vi "Publish Camera Settings.vi"(8 "error in (no error)":errorcluster, 10 "Camera Settings":variant, 11 "IMAQdx Actor in":refnum<class "IMAQdx Actor.lvclass">) -> (0 "error out":errorcluster, 3 "IMAQdx Actor out":refnum<class "IMAQdx Actor.lvclass">)   [LabVIEW 2020, in "IMAQdx Actor.lvlib" / "IMAQdx Actor.lvclass"]
uses:
  IMAQdx Actor.lvclass
  C:/Users/AlexK/work/LabVIEW Programme/POLARIS CAM Log Abw und E/Submodules/HIJ Vision/Camera Actors/Camera Actor/Camera Actor/Camera Actor.lvclass
  IMAQdx Actor.lvclass/IMAQdx Actor.ctl
  Camera Actor/Camera Actor/Camera Actor.lvclass/Camera Actor.ctl
  Camera Actor/Camera Actor/Read Parameter Filter.vi
  Camera Actor/Camera Actor/Camera Actor.lvclass
  <vilib>/vision/driver/NI_Vision_Acquisition_Software.lvlib
  <resource>/objmgr/imaqdx.rc
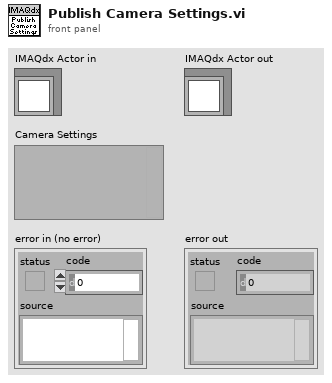
[diagram p1: front panel]
types:
  T1 = typedef "Camera Actor.lvlib/Camera Actor.lvclass/Parameter Filters.ctl" = cluster{"Filter":string[], "Exclude strings":string[]}
  T2 = typedef "IMAQdx.ctl" = refnum<k21>
  T3 = typedef "NI_Vision_Acquisition_Software.lvlib/IMAQdx Attribute Type.ctl" = enum32{"U32", "I64", "DBL", "String", "Enum", "Bool", "Command"}
  T4 = cluster{"Attribute Type":T3, "Readable":bool, "Writable":bool, "Attribute Name":string}[]
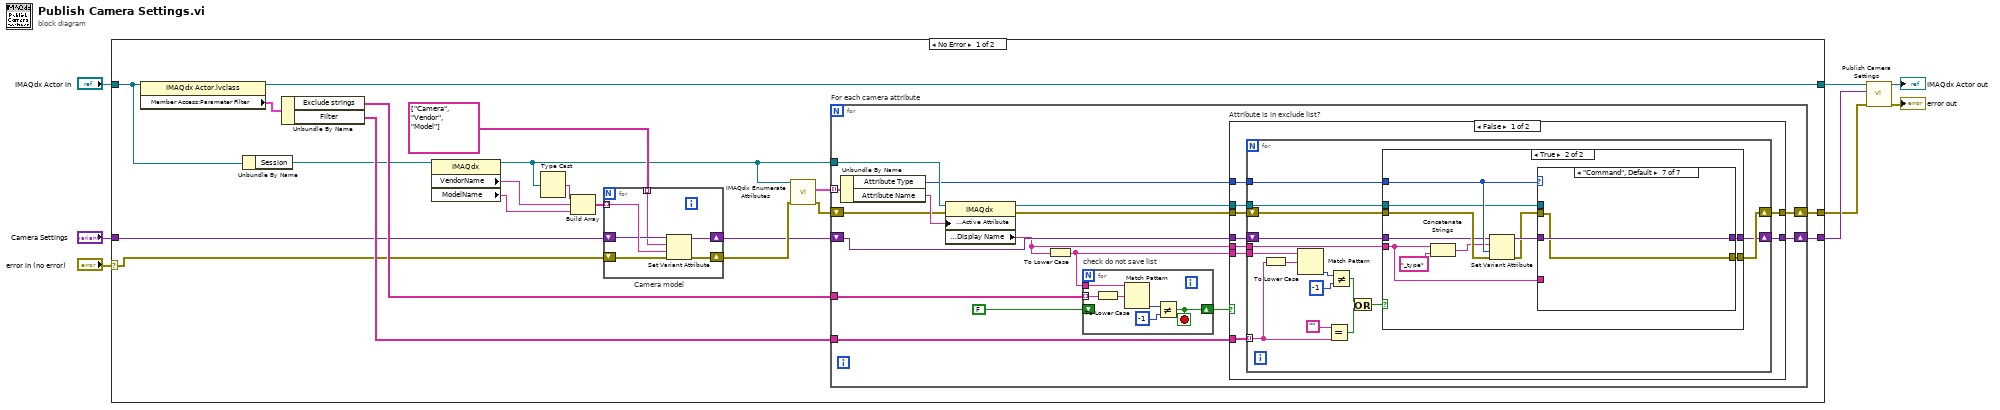
[diagram p0: block diagram]
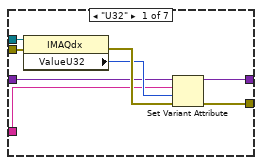
[diagram p3: hidden frame]
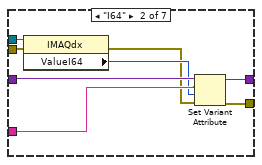
[diagram p4: hidden frame]
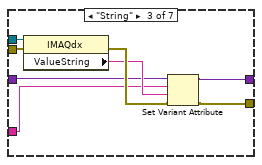
[diagram p5: hidden frame]
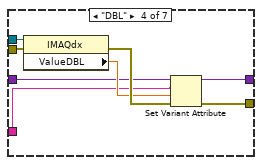
[diagram p6: hidden frame]
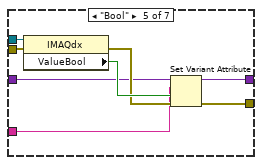
[diagram p7: hidden frame]
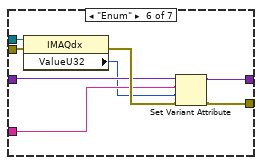
[diagram p8: hidden frame]
diagram:
  n1 = case shown="No Error" "error in (no error)" {
    selector: "error in (no error)" -> [w22 w149]
    tunnel: [w23 w149] -> w1
    tunnel: [w12 w148] -> w4
    tunnel: "IMAQdx Actor in" -> [w10 w148]
    tunnel: "Camera Settings" -> [w9 w147]
    tunnel: [w25 w147] -> w2
    frame No Error {
      n2 = property class="IMAQdx Actor.lvclass"(reference=w10) -> (reference out=w12:refnum<class "IMAQdx Actor.lvclass">, "Member Access:Parameter Filter"=w11:T1)  [unwired: 1 in, 1 out]
      n3 = Unbundle By Name(w10) -> ("Session"=w15:T2)
      n4 = Unbundle By Name(w11) -> ("Exclude strings"=w28:string[], "Filter"=w27:string[])
      n5 = property class="IMAQdx"(reference=w15) -> (reference out=w14:T2, "VendorName"=w21:string, "ModelName"=w20:string)  [unwired: 1 in, 1 out]
      n6 = Type Cast(x=w14) -> (*(type *) &x=w19:string)  [unwired: 1 in]
      n7 = Build Array(w19, w21, w20) -> (w18:string[])
      n8 = for "Camera model" {
        shift-right: [w31] -> w17
        shift-left: w22 -> [w34]
        shift-right: [w33] -> w13
        shift-left: w9 -> [w30]
        tunnel: w18 -> [w32] mode=indexing
        tunnel: string[] ["Camera", "Vendor", "Model"] -> [w29] mode=indexing
        n9 = Set Variant Attribute(Variant=w30, name=w29, value=w32, error in=w34) -> (Variant out=w33:variant, error out=w31:errorcluster)  [unwired: 1 out]
      }
      n10 = call <vilib>:"IMAQdx Enumerate Attributes.vi"("error in"=w17, "Session In"=w14) -> ("error out"=w24:errorcluster, "Attribute Information Array"=w26:T4)  [unwired: 7 in, 1 out]
      n11 = for "For each camera attribute" {
        tunnel: w27 -> [w49]
        tunnel: w26 -> [w50] mode=indexing
        tunnel: w14 -> [w48]
        shift-right: [w44] -> w25
        shift-left: w13 -> [w45]
        shift-right: [w41] -> w23
        shift-left: w24 -> [w40]
        tunnel: w28 -> [w38]
        n12 = Unbundle By Name(w50) -> ("Attribute Type"=w46:T3, "Attribute Name"=w47:string)
        n13 = property class="IMAQdx"(reference=w48, error in=w40, "Camera Attributes:Active Attribute"=w47) -> (reference out=w42:T2, error out=w43:errorcluster, "Camera Attributes:Display Name"=w39:string)
        n14 = To Lower Case(string=w39) -> (all lower case string=w35:string)
        n15 = for "check do not save list" {
          tunnel: w38 -> [w146] mode=indexing
          shift-right: [w143] -> w36
          shift-left: FALSE -> [_]
          tunnel: w35 -> [w141]
          stop <- w143 stop-if-true
          n16 = To Lower Case(string=w146) -> (all lower case string=w142:string)
          n17 = Match Pattern(string=w141, regular expression=w142) -> (offset past match=w145:i32)  [unwired: 1 in, 3 out]
          n18 = Not Equal?(x=w145, y=-1) -> (x != y?=w143:bool)
        }
        n19 = case "Attribute is in exclude list?" shown="False" w36 {
          tunnel: w49 -> [w59 _]
          tunnel: w46 -> [w58 _]
          tunnel: w45 -> [w57 w140]
          tunnel: [w56 w140] -> w44
          tunnel: w43 -> [w55 w139]
          tunnel: w42 -> [w54 _]
          tunnel: [w53 w139] -> w41
          tunnel: w39 -> [w52 _]
          tunnel: w35 -> [w51 _]
          frame False {
            n20 = for {
              tunnel: w59 -> [w67] mode=indexing
              tunnel: w52 -> [w68]
              tunnel: w58 -> [w69]
              shift-right: [w60] -> w56
              shift-left: w57 -> [w66]
              tunnel: w54 -> [w65]
              shift-right: [w63] -> w53
              shift-left: w55 -> [w64]
              tunnel: w51 -> [w61]
              n21 = To Lower Case(string=w67) -> (all lower case string=w75:string)
              n22 = Match Pattern(string=w61, regular expression=w75) -> (offset past match=w71:i32)  [unwired: 1 in, 3 out]
              n23 = Equal?(x="", y=w67) -> (x = y?=w73:bool)
              n24 = Not Equal?(x=w71, y=-1) -> (x != y?=w74:bool)
              n25 = Or(x=w74, y=w73) -> (x .or. y?=w62:bool)
              n26 = case shown="True" w62 {
                tunnel: w69 -> [_ w87]
                tunnel: w68 -> [_ w80]
                tunnel: w66 -> [w77 w86]
                tunnel: [w77 w85] -> w60
                tunnel: w65 -> [_ w84]
                tunnel: w64 -> [w76 w88]
                tunnel: [w76 w83] -> w63
                frame False {
                }
                frame True {
                  n27 = Concatenate Strings(w80, "_type" ("string")) -> (w81:string)
                  n28 = Set Variant Attribute(Variant=w86, name=w81, value=w87, error in=w88) -> (Variant out=w82:variant, error out=w78:errorcluster)  [unwired: 1 out]
                  n29 = case shown="\"Command\", Default" w87 {
                    tunnel: w80 -> [w89 w100 w105 w114 w121 w130 _]
                    tunnel: w82 -> [w90 w99 w107 w113 w122 w131 w138]
                    tunnel: [w91 w102 w106 w120 w128 w132 w138] -> w85
                    tunnel: w84 -> [w94 w104 w110 w119 w127 w136 _]
                    tunnel: w78 -> [w93 w103 w109 w118 w126 w135 w137]
                    tunnel: [w92 w101 w108 w117 w124 w133 w137] -> w83
                    frame "U32" {
                      n30 = property class="IMAQdx"(reference=w94, error in=w93) -> (error out=w96:errorcluster, "ValueU32"=w95:u32)  [unwired: 1 out]
                      n31 = Set Variant Attribute(Variant=w90, name=w89, value=w95, error in=w96) -> (Variant out=w91:variant, error out=w92:errorcluster)  [unwired: 1 out]
                    }
                    frame "I64" {
                      n32 = property class="IMAQdx"(reference=w104, error in=w103) -> (error out=w97:errorcluster, "ValueI64"=w98:i64)  [unwired: 1 out]
                      n33 = Set Variant Attribute(Variant=w99, name=w100, value=w98, error in=w97) -> (Variant out=w102:variant, error out=w101:errorcluster)  [unwired: 1 out]
                    }
                    frame "String" {
                      n34 = property class="IMAQdx"(reference=w110, error in=w109) -> (error out=w112:errorcluster, "ValueString"=w111:string)  [unwired: 1 out]
                      n35 = Set Variant Attribute(Variant=w107, name=w105, value=w111, error in=w112) -> (Variant out=w106:variant, error out=w108:errorcluster)  [unwired: 1 out]
                    }
                    frame "DBL" {
                      n36 = property class="IMAQdx"(reference=w119, error in=w118) -> (error out=w116:errorcluster, "ValueDBL"=w115:dbl)  [unwired: 1 out]
                      n37 = Set Variant Attribute(Variant=w113, name=w114, value=w115, error in=w116) -> (Variant out=w120:variant, error out=w117:errorcluster)  [unwired: 1 out]
                    }
                    frame "Bool" {
                      n38 = property class="IMAQdx"(reference=w127, error in=w126) -> (error out=w123:errorcluster, "ValueBool"=w125:bool)  [unwired: 1 out]
                      n39 = Set Variant Attribute(Variant=w122, name=w121, value=w125, error in=w123) -> (Variant out=w128:variant, error out=w124:errorcluster)  [unwired: 1 out]
                    }
                    frame "Enum" {
                      n40 = property class="IMAQdx"(reference=w136, error in=w135) -> (error out=w134:errorcluster, "ValueU32"=w129:u32)  [unwired: 1 out]
                      n41 = Set Variant Attribute(Variant=w131, name=w130, value=w129, error in=w134) -> (Variant out=w132:variant, error out=w133:errorcluster)  [unwired: 1 out]
                    }
                    frame "Command", Default {
                    }
                  }
                }
              }
            }
          }
          frame True {
          }
        }
      }
    }
    frame Error {
    }
  }
  n42 = call-parent "Publish Camera Settings.vi"("error in (no error)"=w1, "Camera Settings"=w2, "Camera Actor in"=w4) -> ("error out"=→"error out":errorcluster, "Camera Actor out"=→"IMAQdx Actor out":refnum<class "IMAQdx Actor.lvclass">)  [unwired: 7 in]
